vi "Pass_Fail.vi"(8 "error in (no error)":errorcluster, 10 "OK":bool, 11 "Byte Stream File in":refnum<file>) -> (0 "error out":errorcluster, 3 "Byte Stream File out":refnum<file>)   [LabVIEW 2018]
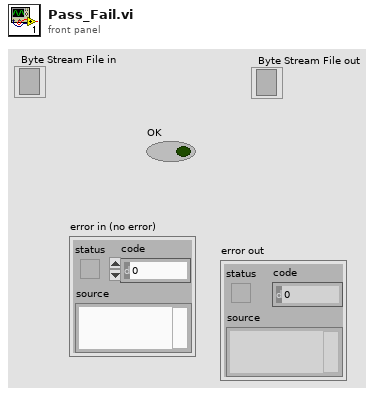
[diagram p1: front panel]
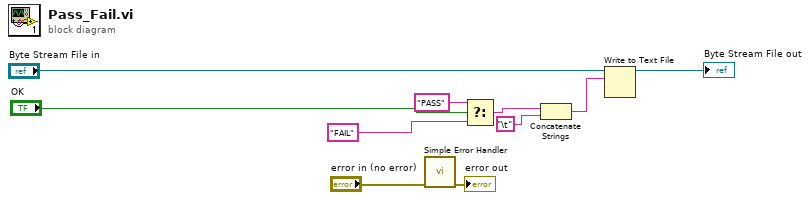
[diagram p0: block diagram]
diagram:
  n1 = call <vilib>:"Simple Error Handler.vi"("error in (no error)"="error in (no error)") -> ("error out"=→"error out":errorcluster)  [unwired: 4 in, 4 out]
  n2 = Select(t="PASS", s="OK", f="FAIL") -> (s? t:f=w8:string)
  n3 = Concatenate Strings(w8, "\t") -> (w6:string)
  n4 = Write to Text File(file (use dialog)="Byte Stream File in", text=w6) -> (refnum out=→"Byte Stream File out":refnum<file>)  [unwired: 2 in, 2 out]
